vi "WPI_SolenoidGet.vi"   [LabVIEW 2017]
doc: "Returns the current value of the solenoid.\n\nThis software is licensed. Open the labview\\readme\\WPI Robotics Library Open Source License.txt file for more information."
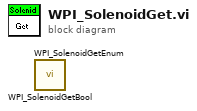
[diagram p0: block diagram]
diagram:
  n1 = call <vilib>:"WPI_SolenoidGetBool.vi"() -> ()  [unwired: 9 in, 3 out]
  n2 = call <vilib>:"WPI_SolenoidGetEnum.vi"() -> ()  [unwired: 9 in, 3 out]
